vi "APS wait multiple int.vi"(7 "Time_Out":i32, 8 "error in (no error)":errorcluster caption="错误输入（无错误）", 9 "Wait_All":i32, 10 "Int_No_Array":i32, 11 "Int_Count":i32) -> (0 "error out":errorcluster caption="错误输出", 2 "Int_No_Array out":i32, 3 "function return":i32)   [LabVIEW 2011, in "APS168.lvlib"]
doc: "I32 FNTYPE APS_wait_multiple_int( I32 Int_Count, I32 *Int_No_Array, I32 Wait_All, I32 Time_Out );"
uses:
  APS168.lvlib
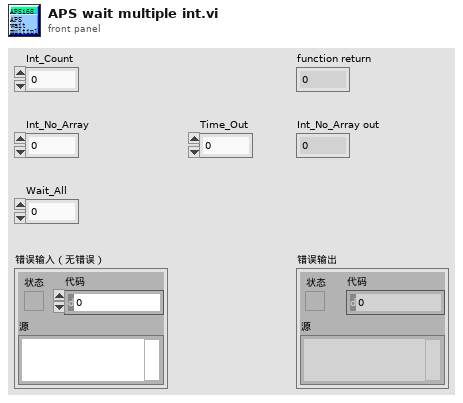
[diagram p1: front panel]
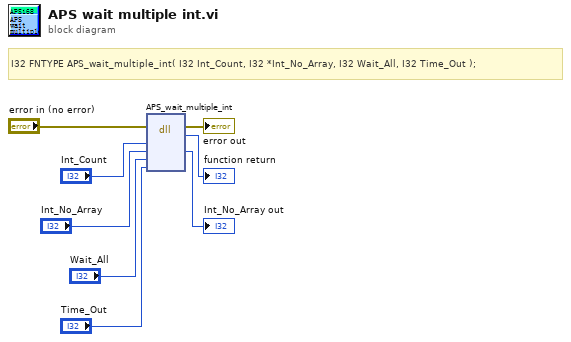
[diagram p0: block diagram]
diagram:
  # "I32 FNTYPE APS_wait_multiple_int( I32 Int_Count, I32 *Int_No_Array, I32 Wait_All, I32 Time_Out );"
  n1 = dll-call lib="PTH1Labs E软件ADLINK 204CAPS_1_7_1_LIB line 连续运动204APS168.*" fn="APS_wait_multiple_int"(error in="error in (no error)", "Int_Count"="Int_Count", "Int_No_Array"="Int_No_Array", "Wait_All"="Wait_All", "Time_Out"="Time_Out") -> (error out=→"error out":errorcluster, →"function return":i32, "Int_No_Array"=→"Int_No_Array out":i32)  [unwired: 5 in, 1 out]
